vi "Write Channel info.vi"(8 "error in":errorcluster, 10 "channel info":T1, 11 "channel in":refnum<class "channel node.lvclass">) -> (0 "error out":errorcluster, 3 "channel out":refnum<class "channel node.lvclass">)   [LabVIEW 2014, in "channel node.lvclass"]
uses:
  channel node.lvclass
  channel configuration/ChannelData.ctl
  channel node.lvclass/channel node.ctl
  channel configuration/channel configuration.lvclass/channel configuration.ctl
  channel configuration/channel configuration.lvclass
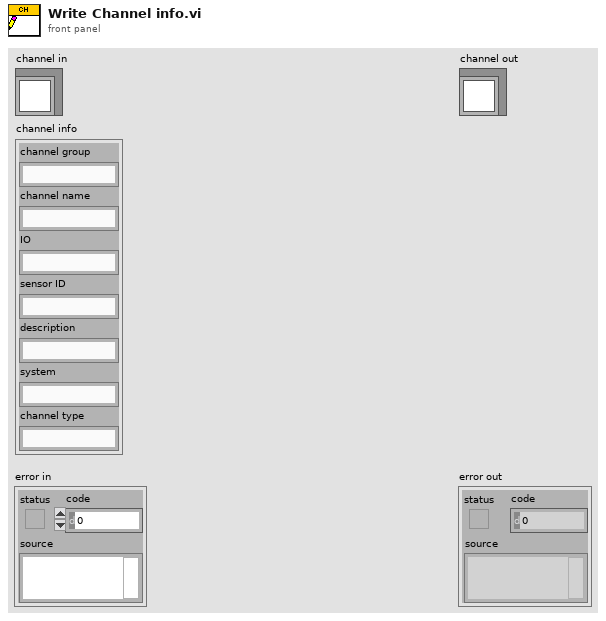
[diagram p1: front panel]
types:
  T1 = typedef "channel configuration.lvclass/ChannelData.ctl" = cluster{"channel group":string, "channel name":string, "IO":string, "sensor ID":string, "description":string, "system":string, "channel type":string}
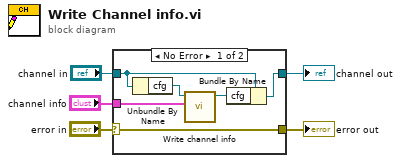
[diagram p0: block diagram]
diagram:
  n1 = case shown="No Error" "error in" {
    selector: "error in" -> [w11 w12]
    tunnel: [w11 w12] -> w4
    tunnel: [w10 w13] -> w2
    tunnel: "channel in" -> [w9 w13]
    tunnel: "channel info" -> [w7 _]
    frame No Error {
      n2 = Unbundle By Name(w9) -> ("cfg"=w8:refnum<class "channel configuration.lvclass">)
      n3 = call "Write channel info.vi"("channel"=w7, "channel config object in"=w8) -> ("channel config object out"=w6:refnum<class "channel configuration.lvclass">)  [unwired: 8 in, 1 out]
      n4 = Bundle By Name(cluster=w9, "cfg"=w6) -> (w10:refnum<class "channel node.lvclass">)
    }
    frame Error {
    }
  }
  "error out" <- w4
  "channel out" <- w2
